vi "Parse Lease ID.vi"(11 "String":string) -> (3 "Lease id":string)   [LabVIEW 2015, in "NI_Azure_Blob.lvlib"]
uses:
  NI_Azure_Blob.lvlib
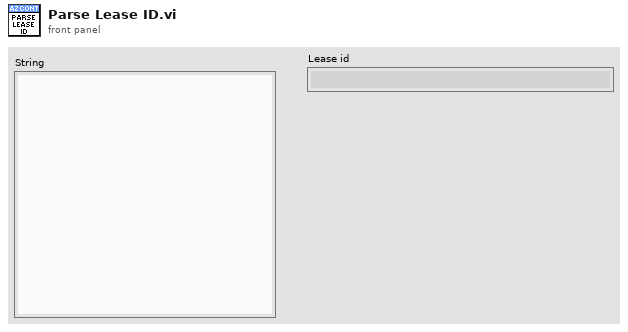
[diagram p1: front panel]
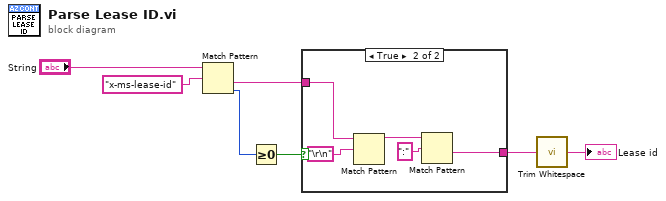
[diagram p0: block diagram]
diagram:
  n1 = Match Pattern(string="String", regular expression="x-ms-lease-id") -> (after substring=w4:string, offset past match=w5:i32)  [unwired: 1 in, 2 out]
  n2 = Greater Or Equal To 0?(x=w5) -> (x >= 0?=w3:bool)
  n3 = case shown="True" w3 {
    tunnel: w4 -> [_ w12]
    tunnel: [_ w8] -> w2
    frame False {
    }
    frame True {
      n4 = Match Pattern(string=w12, regular expression="\r\n") -> (before substring=w10:string)  [unwired: 1 in, 3 out]
      n5 = Match Pattern(string=w10, regular expression=":") -> (after substring=w8:string)  [unwired: 1 in, 3 out]
    }
  }
  n6 = call <vilib>:"Trim Whitespace.vi"("string"=w2) -> ("trimmed string"=→"Lease id":string)  [unwired: 1 in]
